vi "陀螺当量.vi"(11 "x":dbl) -> (3 "子数组":u8[](array[numeric]))   [LabVIEW 2012]
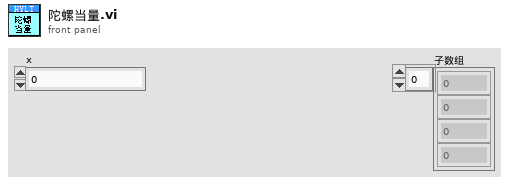
[diagram p1: front panel]
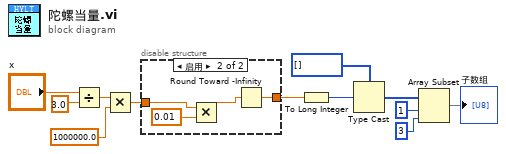
[diagram p0: block diagram]
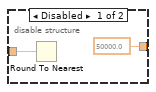
[diagram p2: hidden frame]
diagram:
  n1 = Divide(x="x", y=3.0) -> (x/y=w11:dbl)
  n2 = Multiply(x=w11, y=1000000.0) -> (x*y=w2:dbl)
  n3 = disable-structure shown="启用" {
    disable-tunnel: w2 -> [w14 w17]
    disable-tunnel: [50000.0 w18] -> w1
    frame Disabled {
      n4 = Round To Nearest(number=w14) -> ()  [unwired: 1 out]
    }
    frame Enabled {
      n5 = Multiply(x=w17, y=0.01) -> (x*y=w16:dbl)
      n6 = Round Toward -Infinity(1:w16) -> (0:w18:dbl)
    }
  }
  n7 = To Long Integer(number=w1) -> (32bit integer=w9:i32)
  n8 = Type Cast(type=u8[] [], x=w9) -> (*(type *) &x=w6:u8[])
  n9 = Array Subset(array=w6, index=1 ("索引"), length=3 ("长度")) -> (→"子数组":u8[])
